vi "Teleop Elevator Control.vi"(8 "Button Cluster":T1, 9 "Driver Joystick":T2, 11 "Manipulator Joystick":T2) -> ()   [LabVIEW 2014]
uses:
  <vilib>/Rock Robotics/WPI/Joystick/WPI_JoystickDevRef.ctl
  <vilib>/Rock Robotics/WPI/Joystick/WPI_JoystickDeviceEnum.ctl
  Real-Life Controls/Button Cluster.ctl
  Elevator Control Command.ctl
  Elevator Command.ctl
  Common Code/Elevator Mode.ctl
  Common Code/Elevator Idle Mode.ctl
  Common Code/Elevator State.ctl
  Common Code/Change Detect Int.vi
  Common Code/Change Detect Boolean.vi
  Robot Global Data.vi
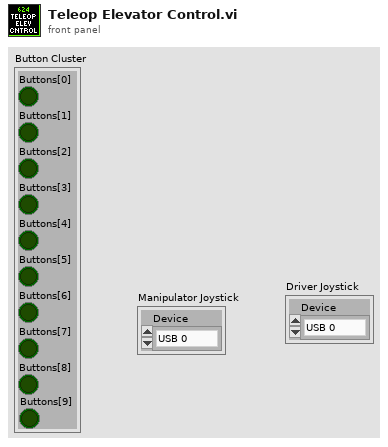
[diagram p1: front panel]
types:
  T1 = typedef "Button Cluster.ctl" = cluster{"Buttons[0]":bool, "Buttons[1]":bool, "Buttons[2]":bool, "Buttons[3]":bool, "Buttons[4]":bool, "Buttons[5]":bool, "Buttons[6]":bool, "Buttons[7]":bool, "Buttons[8]":bool, "Buttons[9]":bool}
  T2 = typedef "WPI_JoystickDevRef.ctl" = cluster{"Device":T3}
  T3 = typedef "WPI_JoystickDeviceEnum.ctl" = enum16{"USB 0", "USB 1", "USB 2", "USB 3", "USB 4", "USB 5"}
  T4 = enum16{"0", "1", "2", "3", "4", "5", "6", "7", "8", "9", "A", "B", "C", "D", "E", "F", "G", "H", "I", "J", "K", "L", "M", "N", "O", "P", "Q", "R", "S", "T", "U", "V", "W", "X", "Y", "Z", "F1", "F2", "F3", "F4", "F5", "F6", "F7", "F8", "F9", "F10", "F11", "F12", "F13", "F14", "F15", "ADD", "BACK", "BACKSLASH", "CAPITAL", "COMMA", "DECIMAL", "DELETE", "DIVIDE", "DOWN", "END", "EQUALS", "ESCAPE", "GRAVE (`)", "HOME", "INSERT", "LBRACKET", "LCONTROL", "LEFT", "L ALT", "LSHIFT", "LWIN", "MINUS", "MULTIPLY", "NEXT", "NUMLOCK", "NUMPAD_0", "NUMPAD_1", "NUMPAD_2", "NUMPAD_3", "NUMPAD_4", "NUMPAD_5", "NUMPAD_6", "NUMPAD_7", "NUMPAD_8", "NUMPAD_9", "PAUSE", "PERIOD", "PRIOR (PG UP)", "RBRACKET", "RCONTROL", "RETURN", "RIGHT", "R ALT", "RSHIFT", "RWIN", "SCROLL", "SEMICOLON", "SLASH", "SPACE", "SUBTRACT", "TAB", "UP", "ENTER (num pad)", "' (quote)"}
  T5 = typedef "Elevator Control Command.ctl" = cluster{"Command":T6, "Manual Motor Out":dbl, "Manual Eject Piston":bool, "Mode":T7, "Override Limits":bool, "Manual Stabilizer":bool, "Manual Finger":bool, "Store Trashcan?":bool, "Hold Low?":bool, "Idle Mode":T8, "HP Load":bool}
  T6 = typedef "Elevator Command.ctl" = enum16{"Idle", "Load 1", "Load 2", "Load 3", "Drop Stack", "Eject Stack", "Untip Trashcan", "Load Trashcan", "HP Load", "HP Score"}
  T7 = typedef "Elevator Mode.ctl" = enum16{"Manual", "Safe", "Auto"}
  T8 = typedef "Elevator Idle Mode.ctl" = enum16{"Load 1", "Load 2", "Load 3", "Load Can", "Untip Can", "Step Load", "Drop Stack"}
  T9 = typedef "Elevator Status.ctl" = cluster{"Height":dbl, "Enc Value":dbl, "Limit Override":bool, "Mode":T7, "High IR":bool, "Motor Out":dbl, "Ping Detect":bool, "Auto Elevator Indicators":T10, "Master Current":dbl, "Slave Current":dbl, "High Current":bool, "Current Tripped":bool, "Top Limit":bool, "Bottom Limit":bool, "Eject Piston":bool, "Stabilizer":bool, "Finger":bool, "Finger Height":dbl, "Finger Raw":dbl}
  T10 = typedef "Auto Elevator Indicators.ctl" = cluster{"Target Out":dbl, "Storing Trashcan?":bool, "State":T11, "In Range":bool, "Store Can Command":bool, "HP Load":bool}
  T11 = typedef "Elevator State.ctl" = enum16{"Idle", "Goto Load Position", "Wait for Load", "Load Drop", "Load Lift", "Drop Stack", "Goto Eject Position", "Eject ", "Raise Trashcan", "Open Stabilizer", "Untip Drop", "Untip Wait", "Untip Lift", "Abort Load", "HP Load Wait", "HP Load Drop", "HP Load Lift", "HP Load Abort", "Close Stabilizer", "HP Load Lift First Tote", "HP Load Drop First Tote", "HP Load Finish"}
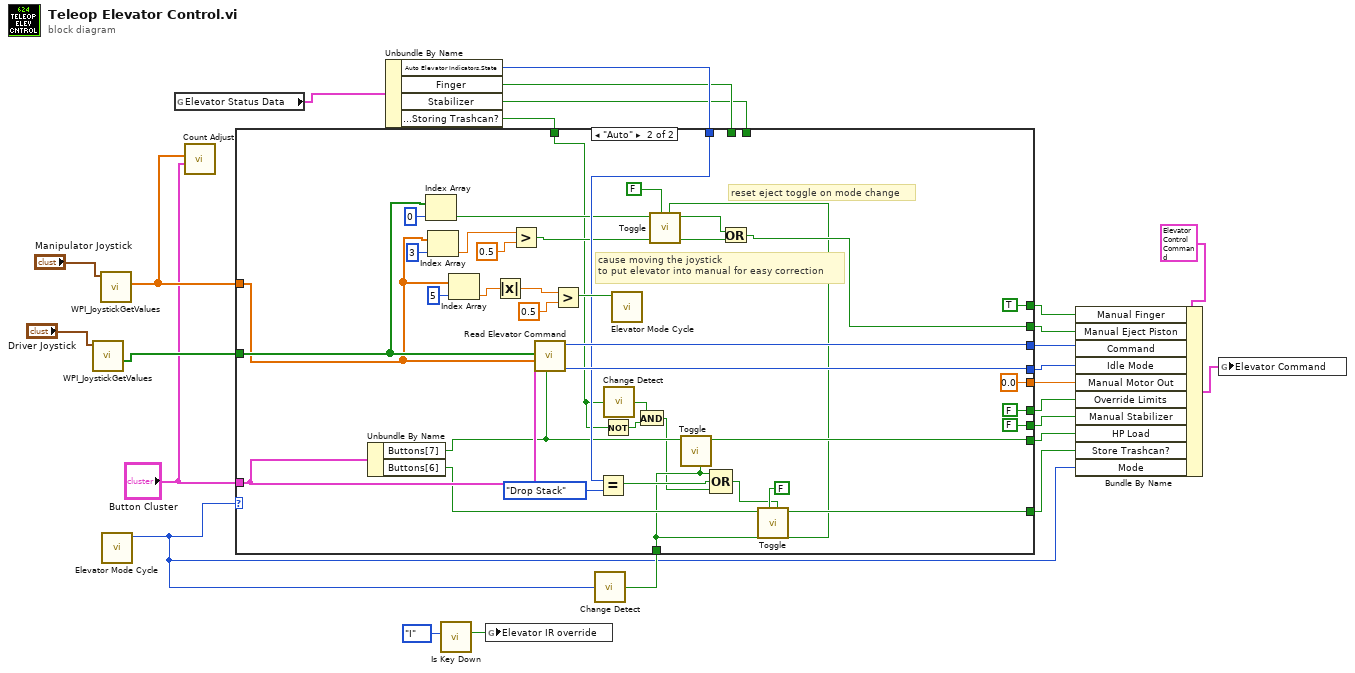
[diagram p0: block diagram]
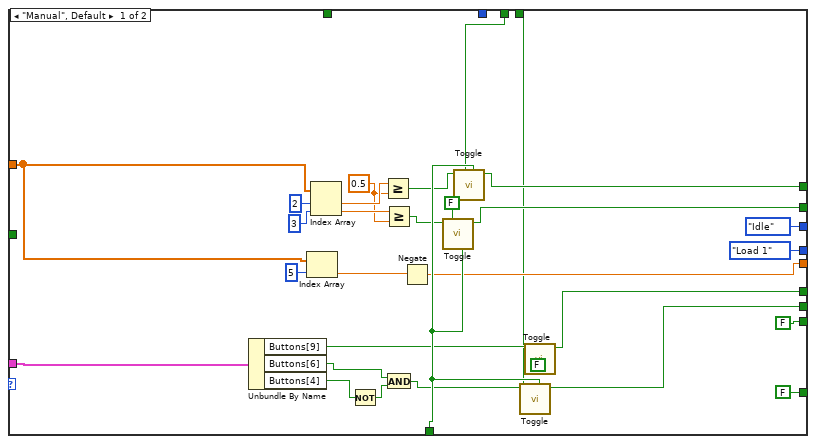
[diagram p2: hidden frame]
diagram:
  n1 = call <vilib>:"WPI_JoystickGetValues.vi"("JoystickDevRef"="Driver Joystick") -> ("Buttons"=w12:bool[])  [unwired: 6 in, 4 out]
  n2 = call <vilib>:"WPI_JoystickGetValues.vi"("JoystickDevRef"="Manipulator Joystick") -> ("Axes"=w8:dbl[])  [unwired: 6 in, 4 out]
  n3 = call "Elevator Mode Cycle.vi"() -> ("Mode"=w2:T7)  [unwired: 11 in]
  n4 = global read "Robot Global Data.vi" "Elevator Status Data"() -> (w3:T9)
  n5 = call "Count Adjust.vi"("Button Cluster"="Button Cluster", "Axes"=w8) -> ()  [unwired: 10 in]
  n6 = Unbundle By Name(w3) -> ("Auto Elevator Indicators.State"=w6:T11, "Finger"=w5:bool, "Stabilizer"=w4:bool, "Auto Elevator Indicators.Storing Trashcan?"=w1:bool)
  n7 = call "Is Key Down.vi"("Key"=T4."I") -> ("Key Down?"=w23:bool)  [unwired: 10 in]
  n8 = global write "Robot Global Data.vi" "Elevator IR override"(w23) -> ()
  n9 = call-poly "Change Detect.vi"("In"=w2) -> ("Changed?"=w18:bool)
  n10 = case shown="\"Auto\"" w2 {
    tunnel: "Button Cluster" -> [w45 w89]
    tunnel: w12 -> [_ w85]
    tunnel: w8 -> [w49 w68]
    tunnel: [w55 w64] -> w19
    tunnel: [Elevator_Command."Idle" ("Command") w90] -> w11
    tunnel: [Elevator_Idle_Mode."Load 1" ("Idle Mode") w91] -> w10
    tunnel: [FALSE ("Toggled") w86] -> w13
    tunnel: [w53 TRUE ("Toggled")] -> w21
    tunnel: w18 -> [w54 w61]
    tunnel: w6 -> [_ w76]
    tunnel: [w46 0.0] -> w17
    tunnel: [w42 FALSE ("Toggled")] -> w15
    tunnel: [w43 FALSE ("Toggled")] -> w16
    tunnel: w5 -> [w26 _]
    tunnel: [FALSE ("Toggled") w87] -> w14
    tunnel: w4 -> [w27 _]
    tunnel: w1 -> [_ w56]
    frame "Manual", Default {
      w37 = 0.5 ("y")
      n11 = Unbundle By Name(w45) -> ("Buttons[9]"=w44:bool, "Buttons[6]"=w30:bool, "Buttons[4]"=w31:bool)
      n12 = Index Array(array=w49, index=5) -> (element=w48:dbl)
      n13 = Index Array(array=w49, index #1=2 ("index"), index #2=3 ("index")) -> (element #1=w51:dbl, element #2=w50:dbl)
      n14 = Not(x=w31) -> (.not. x?=w29:bool)
      n15 = Greater Or Equal?(x=w51, y=w37) -> (x >= y?=w52:bool)
      n16 = Greater Or Equal?(x=w50, y=w37) -> (x >= y?=w38:bool)
      n17 = And(x=w30, y=w29) -> (x .and. y?=w28:bool)
      n18 = Negate(x=w48) -> (-x=w46:dbl)
      n19 = call "Toggle.vi"("Reinit?"=w54, "Initial Value"=FALSE, "In"=w38) -> ("Toggled"=w55:bool)  [unwired: 8 in]
      n20 = call "Toggle.vi"("Reinit?"=w54, "Initial Value"=w26, "In"=w52) -> ("Toggled"=w53:bool)  [unwired: 8 in]
      n21 = call "Toggle.vi"("Reinit?"=w54, "Initial Value"=w27, "In"=w28) -> ("Toggled"=w43:bool)  [unwired: 8 in]
      n22 = call "Toggle.vi"("Initial Value"=FALSE, "In"=w44) -> ("Toggled"=w42:bool)  [unwired: 9 in]
    }
    frame "Auto" {
      # "reset eject toggle on mode change"
      # "cause moving the joystick \nto put elevator into manual for easy correction"
      n23 = Unbundle By Name(w89) -> ("Buttons[7]"=w60:bool, "Buttons[6]"=w88:bool)
      n24 = Index Array(array=w85, index=0) -> (element=w66:bool)
      n25 = Index Array(array=w68, index=3) -> (element=w67:dbl)
      n26 = Index Array(array=w68, index=5) -> (element=w70:dbl)
      n27 = Absolute Value(x=w70) -> (abs(x)=w79:dbl)
      n28 = Greater?(x=w67, y=0.5) -> (0:w72:bool)
      n29 = call "Read Elevator Command.vi"("Reset Idle State"=w60, "Button Cluster"=w89, "Axes"=w68, "Driver Buttons"=w85) -> ("Idle Mode"=w91:T8, "Command"=w90:T6)  [unwired: 6 in]
      n30 = Greater?(x=w79, y=0.5) -> (0:w77:bool)
      n31 = Equal?(x=w76, y=Elevator_State."Drop Stack") -> (x = y?=w62:bool)
      n32 = Not(x=w56) -> (.not. x?=w57:bool)
      n33 = call-poly "Change Detect.vi"("In"=w56) -> ("Changed?"=w59:bool)
      n34 = call "Elevator Mode Cycle.vi"("Set to Manual"=w77) -> ()  [unwired: 10 in, 1 out]
      n35 = And(x=w59, y=w57) -> (x .and. y?=w58:bool)
      n36 = call "Toggle.vi"("Reinit?"=w61, "Initial Value"=FALSE, "In"=w66) -> ("Toggled"=w65:bool)  [unwired: 8 in]
      n37 = call "Toggle.vi"("Reinit?"=w61, "In"=w60) -> ("Toggled"=w87:bool)  [unwired: 9 in]
      n38 = Compound Arithmetic op=OR(w61, w62, w58) -> (w63:bool)
      n39 = Or(x=w65, y=w72) -> (x .or. y?=w64:bool)
      n40 = call "Toggle.vi"("Reinit?"=w63, "Initial Value"=FALSE, "In"=w88) -> ("Toggled"=w86:bool)  [unwired: 8 in]
    }
  }
  n41 = Bundle By Name(cluster=T5 {"Command"=enum."Idle", "Manual Motor Out"=0.0, "Manual Eject Piston"=FALSE, "Mode"=enum."Manual", "Override Limits"=FALSE, "Manual Stabilizer"=FALSE, "Manual Finger"=FALSE, "Store Trashcan?"=FALSE, "Hold Low?"=FALSE, "Idle Mode"=enum."Load Can", "HP Load"=FALSE} ("Elevator Command"), "Manual Finger"=w21, "Manual Eject Piston"=w19, "Command"=w11, "Idle Mode"=w10, "Manual Motor Out"=w17, "Override Limits"=w15, "Manual Stabilizer"=w16, "HP Load"=w14, "Store Trashcan?"=w13, "Mode"=w2) -> (w20:T5)
  n42 = global write "Robot Global Data.vi" "Elevator Command"(w20) -> ()
